vi "dfd_TF Validation.vi"(5 "error in (no error)":errorcluster, 7 "denominator":dbl[](array[numeric]) format="%.2f", 8 "numerator":dbl[](array[numeric]) format="%.2f") -> (0 "error out":errorcluster, 2 "validated denominator":dbl[](array[numeric]) format="%.2f", 3 "validated numerator":dbl[](array[numeric]) format="%.2f")   [LabVIEW 2017, in "NI_DigFilterLicensed.lvlib"]
uses:
  <vilib>/addons/Digital Filter Design/NI_DigFilterLicensed.lvlib
  <vilib>/addons/Digital Filter Design/_Misc.llb/dfd_Error Handlers (Single).vi
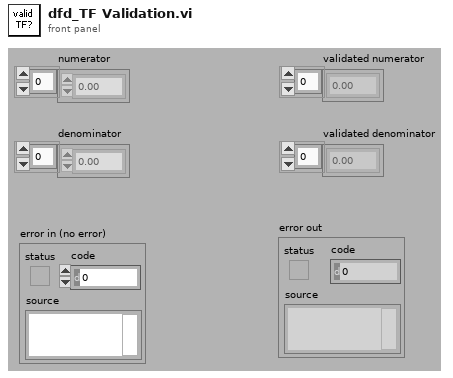
[diagram p1: front panel]
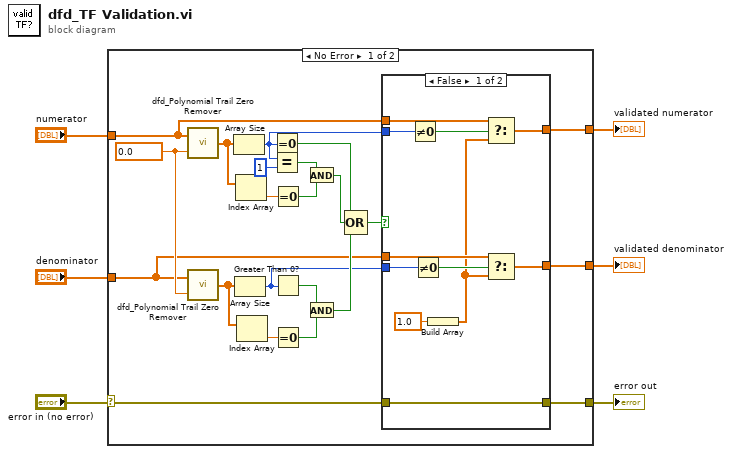
[diagram p0: block diagram]
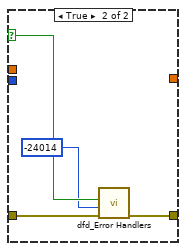
[diagram p2: hidden frame]
diagram:
  n1 = case shown="No Error" "error in (no error)" {
    selector: "error in (no error)" -> [w14 w44]
    tunnel: "numerator" -> [w10 _]
    tunnel: "denominator" -> [w7 _]
    tunnel: [w17 w44] -> w4
    tunnel: [w16 _] -> w3
    tunnel: [w15 _] -> w2
    frame No Error {
      w28 = 0.0 ("tol")
      n2 = call <vilib>:"dfd_Polynomial Trail Zero Remover.vi"("tol"=w28, "poly in"=w10) -> ("poly out"=w9:dbl[])
      n3 = call <vilib>:"dfd_Polynomial Trail Zero Remover.vi"("tol"=w28, "poly in"=w7) -> ("poly out"=w8:dbl[])
      n4 = Array Size(array=w9) -> (size(s)=w12:i32)
      n5 = Array Size(array=w8) -> (size(s)=w13:i32)
      n6 = Index Array(array=w9) -> (element=w27:dbl)  [unwired: 1 in]
      n7 = Index Array(array=w8) -> (element=w24:dbl)  [unwired: 1 in]
      n8 = Equal To 0?(x=w12) -> (x = 0?=w11:bool)
      n9 = Equal?(x=w12, y=1) -> (x = y?=w18:bool)
      n10 = Equal To 0?(x=w27) -> (x = 0?=w26:bool)
      n11 = Greater Than 0?(x=w13) -> (x > 0?=w20:bool)
      n12 = Equal To 0?(x=w24) -> (x = 0?=w25:bool)
      n13 = And(x=w18, y=w26) -> (x .and. y?=w22:bool)
      n14 = And(x=w20, y=w25) -> (x .and. y?=w23:bool)
      n15 = Compound Arithmetic op=OR(w11, w22, w23) -> (w21:bool)
      n16 = case shown="False" w21 {
        selector: w21 -> [_ w41]
        tunnel: w14 -> [w39 w42]
        tunnel: [w39 w43] -> w17
        tunnel: w12 -> [w38 _]
        tunnel: w10 -> [w37 _]
        tunnel: w13 -> [w33 _]
        tunnel: w7 -> [w32 _]
        tunnel: [w30 _] -> w16
        tunnel: [w29 _] -> w15
        frame False {
          n17 = Not Equal To 0?(x=w38) -> (x != 0?=w36:bool)
          n18 = Not Equal To 0?(x=w33) -> (x != 0?=w34:bool)
          n19 = Build Array(1.0 ("element")) -> (w31:dbl[])
          n20 = Select(t=w37, s=w36, f=w31) -> (s? t:f=w30:dbl[])
          n21 = Select(t=w32, s=w34, f=w31) -> (s? t:f=w29:dbl[])
        }
        frame True {
          n22 = call-poly <vilib>:"dfd_Error Handlers.vi"("error in (no error)"=w42, "error code"=-24014 ("ERR_INVALID_TF"), "condition failed?"=w41) -> ("error out"=w43:errorcluster)  [unwired: 8 out]
        }
      }
    }
    frame Error {
    }
  }
  "error out" <- w4
  "validated numerator" <- w3
  "validated denominator" <- w2
